vi "State_Machine.vi"(8 "error in (no error)":errorcluster caption="entrée d'erreur (pas d'erreur)", 11 "Enable_DIO en entrée":refnum<class "Start_Continuous_Ana.lvclass">) -> (0 "error out":errorcluster caption="sortie d'erreur", 2 "Json_String":string, 3 "Enable_DIO en sortie":refnum<class "Start_Continuous_Ana.lvclass">)   [LabVIEW 2020, in "Library Test.lvlib" / "Start_Continuous_Ana.lvclass"]
uses:
  Start_Continuous_Ana.lvclass
  C:/Users/ngarcin/OneDrive - Altyor/Standard TB/Suite TB45/Class/Test/Test (Default)/Test (Default).lvclass
  Commun VI/TypeDef/Variable Printable.ctl
  JSON API/JSON Value/Set from JSON string.vi
  <vilib>/Waveform/WDTOps.llb/WDT Append Waveforms DBL.vi
  Instrument/Instrument (Default)/Class Instrument (Default).lvclass
  JSON API/JSON Value/JSON Value.lvclass
  JSON API/Variant JSON/Variant JSON.lvlib
  JSON API/Get Polymorphic/JSON GetSet.lvlib
  Commun VI/Library Commun.lvlib
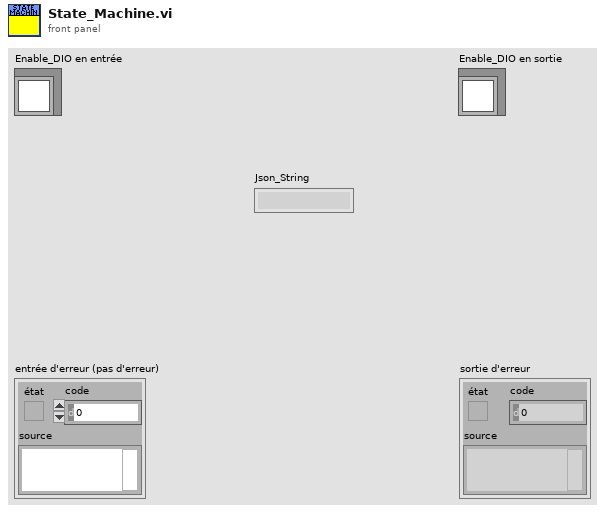
[diagram p1: front panel]
types:
  T1 = typedef "Variable Printable.ctl" = string
  T2 = enum16{"Get Variable", "Get All Variables", "Set Variable", "Delete Variable", "Delete All Variable"}
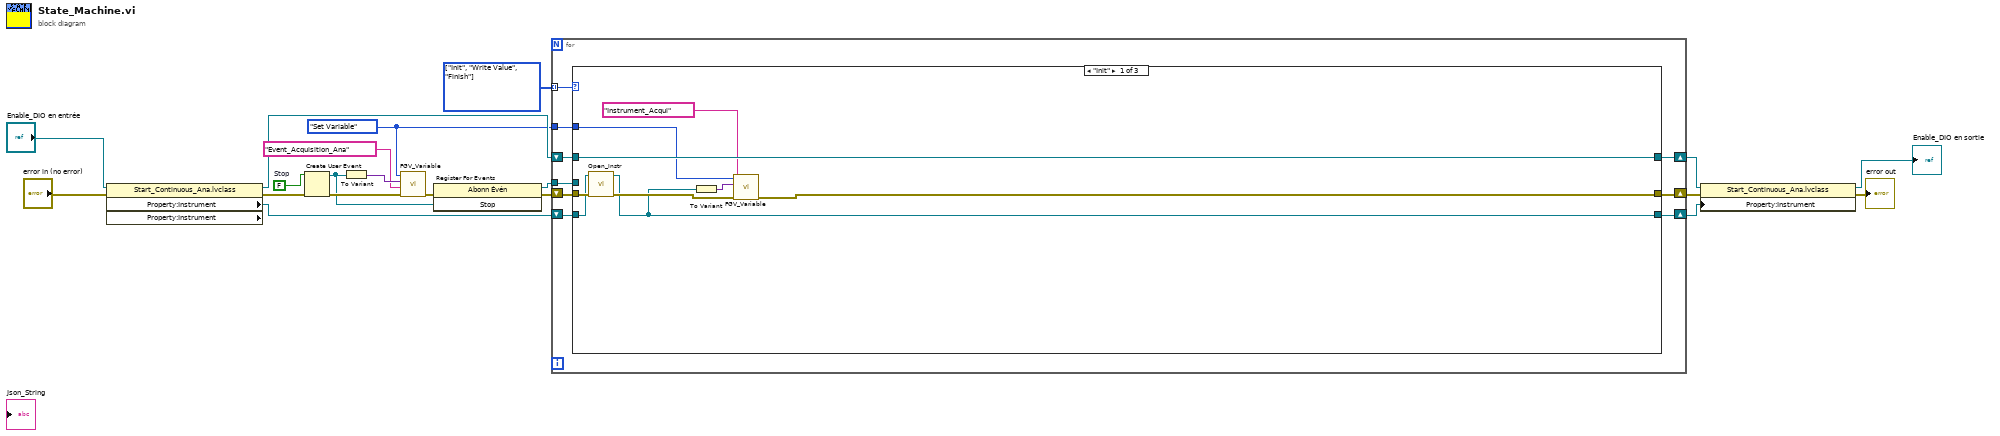
[diagram p0: block diagram]
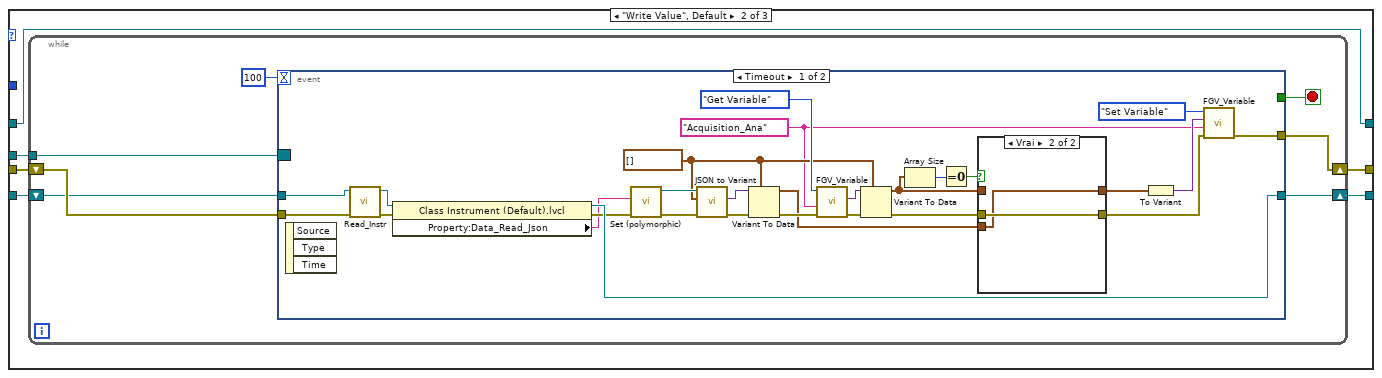
[diagram p2: hidden frame]
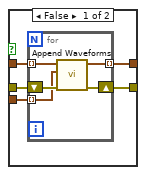
[diagram p3: hidden frame]
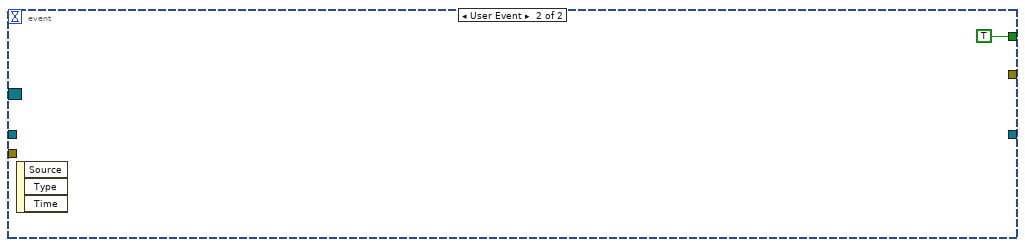
[diagram p4: hidden frame]
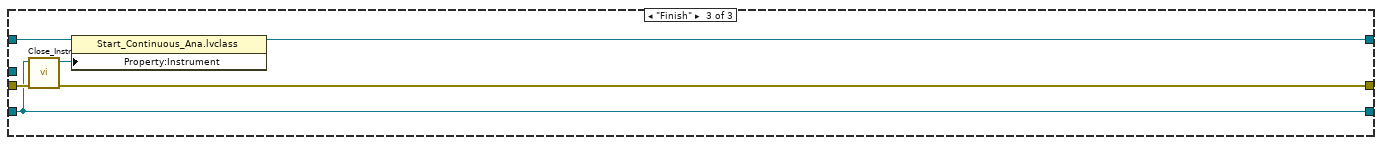
[diagram p5: hidden frame]
diagram:
  w1 = T2."Set Variable" ("Function")
  w10 = FALSE  # Stop
  w19 = enum16{"Init", "Write Value", "Finish"}[] [enum."Init", enum."Write Value", enum."Finish"] items=["Init", "Write Value", "Finish"]
  n1 = property class="Start_Continuous_Ana.lvclass" props=["Property:Instrument", "Property:Instrument"](reference="Enable_DIO en entrée", error in="error in (no error)") -> (reference out=w17:refnum<class "Start_Continuous_Ana.lvclass">, error out=w5:errorcluster, "Property:Instrument"=w18:refnum<class "Class Instrument (Default).lvclass">)  [unwired: 1 out]
  n2 = Create User Event(user event datatype=w10, error in=w5) -> (user event=w3:refnum<user-event>, error out=w4:errorcluster)
  n3 = To Variant(anything=w3) -> (Variant=w7:variant)
  n4 = call "FGV_Variable.vi"("error in (no error)"=w4, "Variable"=T1 "Event_Acquisition_Ana", "Data In"=w7, "Function"=w1) -> ("error out"=w2:errorcluster)  [unwired: 5 in, 2 out]
  n5 = register-events(error in=w2, w3) -> (reference out=w9:refnum<event-registration>, error out=w8:errorcluster)  [unwired: 1 in]
  n6 = for {
    tunnel: w19 -> [w29] mode=indexing
    shift-right: [w27] -> w11
    shift-left: w18 -> [w28]
    shift-right: [w25] -> w14
    shift-left: w17 -> [w26]
    shift-right: [w23] -> w15
    shift-left: w8 -> [w24]
    tunnel: w9 -> [w22]
    tunnel: w1 -> [w21]
    n7 = case shown="\"Init\"" w29 {
      tunnel: w28 -> [w37 w42 w93]
      tunnel: [w31 w41 w93] -> w27
      tunnel: w26 -> [w36 w44 w97]
      tunnel: [w36 w44 w96] -> w25
      tunnel: w24 -> [w38 w43 w95]
      tunnel: [w34 w40 w94] -> w23
      tunnel: w22 -> [_ w39 _]
      tunnel: w21 -> [w33 _ _]
      frame "Init" {
        n8 = call-dynamic "Open_Instr.vi"("error in (no error)"=w38, "Class Multimeter (Default) en entrée"=w37) -> ("error out"=w35:errorcluster, "Class Multimeter (Default) en sortie"=w31:refnum<class "Class Instrument (Default).lvclass">)  [unwired: 8 in]
        n9 = To Variant(anything=w31) -> (Variant=w32:variant)
        n10 = call "FGV_Variable.vi"("error in (no error)"=w35, "Variable"=T1 "Instrument_Acqui", "Data In"=w32, "Function"=w33) -> ("error out"=w34:errorcluster)  [unwired: 5 in, 2 out]
      }
      frame "Write Value", Default {
        n11 = while {
          shift-right: [w48] -> w40
          shift-left: w43 -> [w51]
          shift-right: [w49] -> w41
          shift-left: w42 -> [w50]
          tunnel: w39 -> [w46]
          stop <- w45 stop-if-true
          n12 = event shown="[0] Timeout" {
            selector: w46 -> [_ _]
            dyn-events: _ -> [_ _]
            timeout: 100 -> [_ _]
            tunnel: w51 -> [w78 _]
            tunnel: w50 -> [w77 _]
            tunnel: [w75 _] -> w49
            tunnel: [w60 _] -> w48
            tunnel: [_ TRUE] -> w45
            event Timeout {
              w55 = T1 "Acquisition_Ana" ("Variable")
              w63 = waveform(dbl)[] [] ("data")
              n13 = event-data() -> ()  [unwired: 1 in, 3 out]
              n14 = call-dynamic "Read_Instr.vi"("error in (no error)"=w78, "Class Instrument (Default) en entrée"=w77) -> ("error out"=w74:errorcluster, "Class Instrument (Default) en sortie"=w76:refnum<class "Class Instrument (Default).lvclass">)  [unwired: 8 in]
              n15 = property class="Class Instrument (Default).lvcl"(reference=w76, error in=w74) -> (reference out=w75:refnum<class "Class Instrument (Default).lvclass">, error out=w69:errorcluster, "Property:Data_Read_Json"=w68:string)
              n16 = call-poly "Set (polymorphic).vi"("error in (no error)"=w69, "JSON stream"=w68) -> ("error out"=w72:errorcluster, "JSON Value out"=w70:refnum<class "JSON Value.lvclass">)  [unwired: 7 in, 1 out]
              n17 = call "JSON to Variant.vi"("error in (no error)"=w72, "Variant (Data Type)"=w63, "JSON Value"=w70) -> ("error out"=w71:errorcluster, "Variant out"=w73:variant)  [unwired: 7 in]
              n18 = Variant To Data(error in=w71, type=w63, Variant=w73) -> (data=w56:waveform(dbl)[], error out=w64:errorcluster)
              n19 = call "FGV_Variable.vi"("error in (no error)"=w64, "Variable"=w55, "Function"=T2."Get Variable") -> ("error out"=w66:errorcluster, "Data Out"=w65:variant)  [unwired: 6 in, 1 out]
              n20 = Variant To Data(error in=w66, type=w63, Variant=w65) -> (data=w54:waveform(dbl)[], error out=w62:errorcluster)
              n21 = Array Size(array=w54) -> (size(s)=w53:i32)
              n22 = Equal To 0?(x=w53) -> (x = 0?=w52:bool)
              n23 = case shown="Vrai" w52 {
                tunnel: w62 -> [w83 w90]
                tunnel: [w82 w90] -> w61
                tunnel: [w81 w89] -> w58
                tunnel: w56 -> [w80 w89]
                tunnel: w54 -> [w79 _]
                frame False {
                  n24 = for {
                    tunnel: w79 -> [w88] mode=indexing
                    shift-right: [w86] -> w82
                    shift-left: w83 -> [w87]
                    tunnel: [w85] -> w81 mode=indexing
                    tunnel: w80 -> [w84] mode=indexing
                    n25 = call-poly <vilib>:"Append Waveforms.vi"("error in (no error)"=w87, "waveform B"=w84, "waveform A"=w88) -> ("error out"=w86:errorcluster, "waveform out"=w85:waveform(dbl))  [unwired: 7 in]
                  }
                }
                frame True {
                }
              }
              n26 = To Variant(anything=w58) -> (Variant=w57:variant)
              n27 = call "FGV_Variable.vi"("error in (no error)"=w61, "Variable"=w55, "Data In"=w57, "Function"=T2."Set Variable") -> ("error out"=w60:errorcluster)  [unwired: 5 in, 2 out]
            }
            event User Event {
              n28 = event-data() -> ()  [unwired: 1 in, 3 out]
            }
          }
        }
      }
      frame "Finish" {
        n29 = call-dynamic "Close_Instr.vi"("error in (no error)"=w95, "Class Instrument (Default) en entrée"=w93) -> ("error out"=w94:errorcluster, "Class Instrument (Default) en sortie"=w92:refnum<class "Class Instrument (Default).lvclass">)  [unwired: 8 in]
        n30 = property class="Start_Continuous_Ana.lvclass"(reference=w97, "Property:Instrument"=w92) -> (reference out=w96:refnum<class "Start_Continuous_Ana.lvclass">)  [unwired: 1 in, 1 out]
      }
    }
  }
  n31 = property class="Start_Continuous_Ana.lvclass"(reference=w14, error in=w15, "Property:Instrument"=w11) -> (reference out=→"Enable_DIO en sortie":refnum<class "Start_Continuous_Ana.lvclass">, error out=→"error out":errorcluster)
